vi "ep_Calculate NEMA Derating Factor.vi"(8 "error in (no error)":errorcluster, 11 "NEMA unbalance [%]":dbl) -> (0 "error out":errorcluster, 3 "NEMA unbalance derating factor":dbl format="%#_3f")   [LabVIEW 2014, in "NI_EP_Motor Monitoring.lvlib"]
uses:
  <vilib>/addons/Electrical Power/Motor Monitoring/NI_EP_Motor Monitoring.lvlib
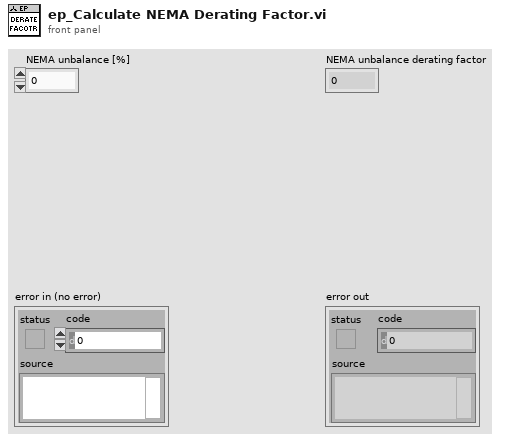
[diagram p1: front panel]
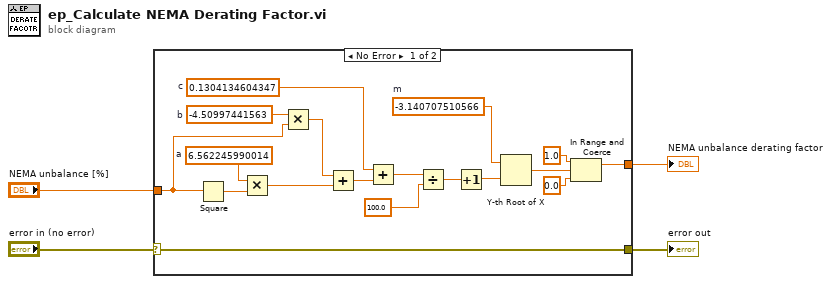
[diagram p0: block diagram]
diagram:
  n1 = case shown="No Error" "error in (no error)" {
    selector: "error in (no error)" -> [w22 w23]
    tunnel: "NEMA unbalance [%]" -> [w11 _]
    tunnel: [w22 w23] -> w2
    tunnel: [w5 _] -> w1
    frame No Error {
      w6 = -3.140707510566  # m
      w13 = 0.1304134604347  # c
      w12 = -4.50997441563  # b
      w15 = 6.562245990014  # a
      n2 = Square(x=w11) -> (x^2=w14:dbl)
      n3 = Multiply(x=w15, y=w14) -> (x*y=w10:dbl)
      n4 = Multiply(x=w12, y=w11) -> (x*y=w9:dbl)
      n5 = Add(x=w9, y=w10) -> (x+y=w8:dbl)
      n6 = Add(x=w13, y=w8) -> (x+y=w7:dbl)
      n7 = Divide(x=w7, y=100.0) -> (x/y=w18:dbl)
      n8 = Increment(x=w18) -> (x+1=w16:dbl)
      n9 = Y-th Root of X(1:w16, 2:w6) -> (0:w19:dbl)
      n10 = In Range and Coerce(upper limit=1.0, x=w19, lower limit=0.0 ("upper limit")) -> (coerced(x)=w5:dbl)  [unwired: 1 out]
    }
    frame Error {
    }
  }
  "NEMA unbalance derating factor" <- w1
  "error out" <- w2
